vi "MaxAndMin.vi"() -> ()   [LabVIEW 2019]
panel:
  out "min(x,y)":dbl
  out "max(x,y)":dbl
  in  "b":dbl
  in  "a":dbl
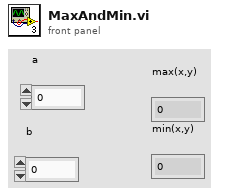
[diagram p1: front panel]
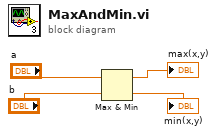
[diagram p0: block diagram]
diagram:
  n1 = Max & Min(x="a", y="b") -> (max(x,y)=→"max(x,y)":dbl, min(x,y)=→"min(x,y)":dbl)
